vi "StepIndex.vi"() -> (1 "StepIndex":string="StepIndex")   [LabVIEW 2016, in "SeqProcessor.lvlib"]
uses:
  SeqProcessor.lvlib
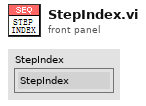
[diagram p1: front panel]
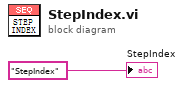
[diagram p0: block diagram]
diagram:
  "StepIndex" <- "StepIndex" ("Tag")
